vi "Update Preview Graph.vi"(11 "UI Data in":refnum<class "Settings UI.lvclass">) -> (3 "UI Data out":refnum<class "Settings UI.lvclass">)   [LabVIEW 2020, in "Output Sequencer.lvlib" / "Settings UI.lvclass"]
uses:
  Settings UI.lvclass
  Settings UI.lvclass/Settings UI.ctl
  Output Sequencer/Output Sequencer.lvclass
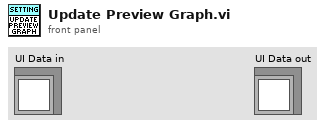
[diagram p1: front panel]
types:
  T1 = typedef "Output Sequencer.lvlib/Settings UI.lvclass/Settings.ctl" = cluster{"Plug-in Version":string, "Step Values":T2[], "Only Execute When Test Running":bool, "Reset Sequence When Test Starts":bool, "Number of Sequence Steps":i32, "Num of Analog Channels":i32, "Num of Digital Channels":i32, "Delay Before Starting Sequence":dbl, "Default Analog Values":dbl[], "Default Digital Values":bool[], "Max Iterations":u32, "Use last value when stopped":bool, "Prioritize exact values":bool, "Enable advanced step timing":bool, "Enable step conditions":bool, "Show confirmation dialogs":bool, "Start condition":string, "Enable re-triggering":bool, "Stop condition":string}
  T2 = typedef "Output Sequencer.lvlib/Settings UI.lvclass/Step Settings.ctl" = cluster{"Description":string, "Precondition":string, "Duration":dbl, "Mode":string, "Delay Between Values":dbl, "Analog Values":string[], "Digital Values":string[], "Postcondition":string, "On True":string, "On False":string}
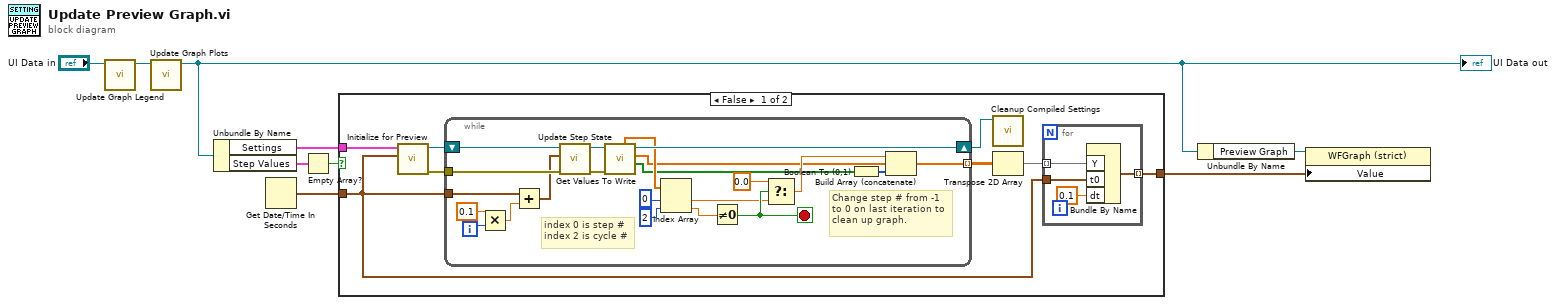
[diagram p0: block diagram]
diagram:
  n1 = call "Update Graph Legend.vi"("UI Data in"="UI Data in") -> ("UI Data out"=w8:refnum<class "Settings UI.lvclass">)  [unwired: 10 in]
  n2 = call "Update Graph Plots.vi"("UI Data in"=w8) -> ("UI Data out"=w1:refnum<class "Settings UI.lvclass">)  [unwired: 10 in]
  "UI Data out" <- w1
  n3 = Unbundle By Name(w1) -> ("Settings"=w3:T1, "Step Values"=w6:T2[])
  n4 = Get Date/Time In Seconds() -> (seconds since 1Jan1904=w4:timestamp)
  n5 = Empty Array?(array=w6) -> (empty?=w5:bool)
  n6 = case shown="False" w5 {
    tunnel: w4 -> [w11 _]
    tunnel: [w15 _] -> w7
    tunnel: w3 -> [w14 _]
    frame False {
      n7 = call "Initialize for Preview.vi"("Current Time"=w11, "Settings"=w14) -> ("error out"=w10:errorcluster, "Plugin out"=w13:refnum<class "Output Sequencer.lvclass">)  [unwired: 8 in]
      n8 = while {
        shift-right: [w30] -> w12
        shift-left: w13 -> [w22]
        tunnel: w11 -> [w37]
        tunnel: [w31] -> w17 mode=indexing
        tunnel: w10 -> [w21]
        i -> [w39]
        stop <- w29 stop-if-true
        # "Change step # from -1\nto 0 on last iteration to\nclean up graph."
        # "index 0 is step #\nindex 2 is cycle #"
        n9 = Multiply(x=0.1, y=w39) -> (x*y=w36:dbl)
        n10 = Add(x=w37, y=w36) -> (x+y=w18:timestamp)
        n11 = call "Update Step State.vi"("error in (no error)"=w21, "Current Time"=w18, "Output Sequencer in"=w22) -> ("error out"=w19:errorcluster, "Output Sequencer out"=w20:refnum<class "Output Sequencer.lvclass">)  [unwired: 6 in, 1 out]
        n12 = call "Get Values To Write.vi"("error in (no error)"=w19, "Output Sequencer in"=w20) -> ("Digital Values to Write"=w23:bool[], "Analog Values to Write"=w24:dbl[], "Output Sequencer out"=w30:refnum<class "Output Sequencer.lvclass">, "Sequence State Channels to Write"=w25:dbl[])  [unwired: 5 in, 1 out]
        n13 = Index Array(array=w25, index #1=0 ("index"), index #2=2 ("index")) -> (element #1=w28:dbl, element #2=w34:dbl)
        n14 = Not Equal To 0?(x=w34) -> (x != 0?=w29:bool)
        n15 = Select(t=0.0, s=w29, f=w28) -> (s? t:f=w26:dbl)
        n16 = Boolean To (0,1)(Boolean=w23) -> (0, 1=w32:i16[])
        n17 = Build Array (concatenate)(w26, w24, w32) -> (w31:dbl[])
      }
      n18 = call "Cleanup Compiled Settings.vi"("Plugin in"=w12) -> ()  [unwired: 9 in, 2 out]
      n19 = Transpose 2D Array(2D array=w17) -> (transposed array=w16:dbl[][])
      n20 = for {
        tunnel: w16 -> [w43] mode=indexing
        tunnel: w11 -> [w42]
        tunnel: [w40] -> w15 mode=indexing
        n21 = Bundle By Name("Y"=w43, "t0"=w42, "dt"=0.1) -> (w40:waveform(dbl))  [unwired: 1 in]
      }
    }
    frame True {
    }
  }
  n22 = Unbundle By Name(w1) -> ("Preview Graph"=w2:refnum<vi>)
  n23 = property class="WFGraph (strict)"(reference=w2, "Value"=w7) -> ()  [unwired: 1 in, 2 out]
